vi "+S2C_Omnia8257_Process.vi"(8 "Error In":errorcluster) -> (0 "Error Out":errorcluster)   [LabVIEW 2015]
uses:
  VIs/S2C_OM8257_Proc_Globals.vi
panel:
  out "Err":bool
  in  "Clear":bool
  out "Exit":bool
  in  "LogDepth":u32=10 caption="Log Depth"
  in  "CtrlTab":T1(tab)
  in  "Init":T2={"P1C1"={"Resource Name"="COM4", "Baud Rate"=57600, "Data Bits"=8, "Parity"=0, "Stop Bits"=10, "Flow Control"=0, "Timeout"=5000, "Reset"=TRUE, "P1C1Exe"=FALSE}} {"P1C1"."Parity" items=["None", "Odd", "Even", "Mark", "Space"]; "P1C1"."Flow Control" items=["None", "XON/XOFF", "RTS/CTS", "XON/XOFF & RTS/CTS", "DTR/DSR", "XON/XOFF & DTR/DSR"]; "P1C1"."Stop Bits" items=["1.0"=10, "1.5"=15, "2.0"=20]; "P1C1"."Data Bits" min=7 max=8 step=1}
  in  "CFG-Step":enum32{"ACW", "LLT", "GND", "RUN", "PROMPT"}(tab)
  in  "ACW":T3={"Voltage (V)"=1240, "High Limit Total (mA)"=10.0, "Low Limit Total (mA)"=0.0, "Ramp Up Time (s)"=0.1, "Dwell Time (s)"=1.0, "Arc Sense"=5, "Arc Detect"=FALSE, "High Limit Real (mA)"=10.0, "Low Limit Real (mA)"=0.0, "Ramp Down Time (s)"=0.0, "Continuity"=FALSE, "Offset (mA)"=0.0, "Auto Offset"=FALSE, "DUT Output"=FALSE, "Frequency (Hz)"=60, "Scanner?"=FALSE, "Step Selection"=1, "Add Step"=FALSE, "ACW-Scan"={"Scan16"=1, "Scan15"=1, "Scan14"=1, "Scan13"=1, "Scan12"=1, "Scan11"=1, "Scan10"=1, "Scan9"=1, "Scan8"=1, "Scan7"=1, "Scan6"=1, "Scan5"=1, "Scan4"=1, "Scan3"=1, "Scan2"=1, "Scan1"=1}, "P1P1C1Exe"=FALSE} caption="CfgStep ACW" {"ACW-Scan"."Scan16" min=0 max=2 step=1 scale=0.0..2.0; "ACW-Scan"."Scan15" min=0 max=2 step=1 scale=0.0..2.0; "ACW-Scan"."Scan14" min=0 max=2 step=1 scale=0.0..2.0; "ACW-Scan"."Scan13" min=0 max=2 step=1 scale=0.0..2.0; "ACW-Scan"."Scan12" min=0 max=2 step=1 scale=0.0..2.0; "ACW-Scan"."Scan11" min=0 max=2 step=1 scale=0.0..2.0; "ACW-Scan"."Scan10" min=0 max=2 step=1 scale=0.0..2.0; "ACW-Scan"."Scan9" min=0 max=2 step=1 scale=0.0..2.0; "ACW-Scan"."Scan8" min=0 max=2 step=1 scale=0.0..2.0; "ACW-Scan"."Scan7" min=0 max=2 step=1 scale=0.0..2.0; "ACW-Scan"."Scan6" min=0 max=2 step=1 scale=0.0..2.0; "ACW-Scan"."Scan5" min=0 max=2 step=1 scale=0.0..2.0; "ACW-Scan"."Scan4" min=0 max=2 step=1 scale=0.0..2.0; "ACW-Scan"."Scan3" min=0 max=2 step=1 scale=0.0..2.0; "ACW-Scan"."Scan2" min=0 max=2 step=1 scale=0.0..2.0; "ACW-Scan"."Scan1" min=0 max=2 step=1 scale=0.0..2.0; "Offset (mA)" format="%.2g"; "Ramp Down Time (s)" format="%.1g"; "Dwell Time (s)" format="%.1g"; "High Limit Real (mA)" format="%.2g"; "Low Limit Total (mA)" format="%.3g"; "High Limit Total (mA)" format="%.2g"; "Low Limit Real (mA)" format="%.3g"; "Ramp Up Time (s)" format="%.1g"}
  in  "LLT":T4={"Leakage-Hi (V)"=6000.0, "Leakage-Lo (V)"=0.0, "Voltage-Hi (V)"=125.0, "Voltage-Lo (V)"=0.0, "Dwell (s)"=0.5, "Delay (s)"=1.0, "Offset (uA)"=10.0, "AC Src Voltage (V)"=115.0, "AC Src A-Hi (A)"=0.0, "AC Source"=FALSE, "AC Src Frequency"=60.0, "Auto Offset"=FALSE, "Reverse"=FALSE, "Active Link"=FALSE, "AC Src OC Fold"=FALSE, "Neutral"=FALSE, "Ground"=FALSE, "Leakage"=FALSE, "Ranging Mode"=FALSE, "AC Src Output"=TRUE, "AC Src Range"=TRUE, "Measure Device"=0, "Probe"=0, "Filter Mode"=0, "Scanner?"=FALSE, "Step Selection"=1, "Add Step"=FALSE, "ACW-Scan"={"Scan16"=1, "Scan15"=1, "Scan14"=1, "Scan13"=1, "Scan12"=1, "Scan11"=1, "Scan10"=1, "Scan9"=1, "Scan8"=1, "Scan7"=1, "Scan6"=1, "Scan5"=1, "Scan4"=1, "Scan3"=1, "Scan2"=1, "Scan1"=1}, "P1P2C1Exe"=FALSE} caption="CfgStep LLT" {"Filter Mode" items=["AC+DC", "AC", "DC"]; "Probe" items=["Ground To Line", "Probe-HI To Line", "Probe-HI To Probe-Lo"]; "Measure Device" items=["UL544NP", "UL544P", "IEC60601 UL2601", "UL1563", "IEC60990 Fig4-U1 IEC60950", "IEC60990 Fig4-U2 IEC60950", "IEC60990 Fig5-U3", "External", "N/A", "Frequency Check"]; "AC Src Frequency" format="%#.6f"; "Offset (uA)" format="%#.2g"; "ACW-Scan"."Scan16" min=0 max=2 step=1 scale=0.0..2.0; "ACW-Scan"."Scan15" min=0 max=2 step=1 scale=0.0..2.0; "ACW-Scan"."Scan14" min=0 max=2 step=1 scale=0.0..2.0; "ACW-Scan"."Scan13" min=0 max=2 step=1 scale=0.0..2.0; "ACW-Scan"."Scan12" min=0 max=2 step=1 scale=0.0..2.0; "ACW-Scan"."Scan11" min=0 max=2 step=1 scale=0.0..2.0; "ACW-Scan"."Scan10" min=0 max=2 step=1 scale=0.0..2.0; "ACW-Scan"."Scan9" min=0 max=2 step=1 scale=0.0..2.0; "ACW-Scan"."Scan8" min=0 max=2 step=1 scale=0.0..2.0; "ACW-Scan"."Scan7" min=0 max=2 step=1 scale=0.0..2.0; "ACW-Scan"."Scan6" min=0 max=2 step=1 scale=0.0..2.0; "ACW-Scan"."Scan5" min=0 max=2 step=1 scale=0.0..2.0; "ACW-Scan"."Scan4" min=0 max=2 step=1 scale=0.0..2.0; "ACW-Scan"."Scan3" min=0 max=2 step=1 scale=0.0..2.0; "ACW-Scan"."Scan2" min=0 max=2 step=1 scale=0.0..2.0; "ACW-Scan"."Scan1" min=0 max=2 step=1 scale=0.0..2.0; "Voltage-Lo (V)" format="%#.2g"; "Voltage-Hi (V)" format="%#.3g"; "Leakage-Lo (V)" format="%#.2g"; "Dwell (s)" format="%.1g"}
  in  "GND":T5={"Current (A)"=1240.0, "Voltage (V)"=10.0, "Hi-Limit (mohm)"=100, "Lo-Limit (mhom)"=0, "Dwell (s)"=1.0, "Offset (mhom)"=0, "Auto Offset"=FALSE, "Frequency (Hz)"=60, "DualCHEK"=0, "Scanner Selection"=0, "Scanner?"=FALSE, "Step Selection"=1, "Add Step"=FALSE, "P1P3C1Exe"=FALSE} caption="CfgStep GND" {"DualCHEK" items=["OFF", "ACW", "DCW"]}
  in  "RUN":T6={"Voltage-Hi (V)"=125.0, "Voltage-Lo (V)"=0.0, "Amp-Hi (A)"=10.0, "Amp-Lo (A)"=0.0, "Dwell (s)"=1.0, "Delay (s)"=0.2, "Leakage-Hi (mA)"=10.0, "Leakage-Lo (mA)"=0.0, "Power-Hi (W)"=1000, "Power-Lo (W)"=0, "PF-Hi"=1.0, "PF-Lo"=0.0, "AC Src Voltage (V)"=115.0, "AC Src A-Hi (A)"=0.0, "AC Source"=FALSE, "AC Src Frequency (Hz)"=60, "AC Src OC Fold"=FALSE, "AC Src Output"=TRUE, "AC Src Range"=TRUE, "Active Link"=FALSE, "Step Selection"=1, "Add Step"=FALSE, "P1P4C1Exe"=FALSE} caption="CfgStep RUN"
  in  "Prompt":cluster{"Prompt":string, "P1P5C1Exe":bool}={"Prompt"="<Enter Prompt>", "P1P5C1Exe"=FALSE} caption="CfgStep Prompt"
  in  "CfgSys":T7
  in  "ActStatus":cluster{"P4C1":cluster{"P4C1Exe":bool}}
  in  "ActFile":T8={"P5C1"={"File Number"=1, "Filename"="<Filename>", "P5C1Exe"=FALSE}, "P5C2"={"File Number"=1, "P5C2Exe"=FALSE}, "P5C3"={"File Number"=1, "P5C3Exe"=FALSE}, "P5C4"={"File Number"=1, "P5C4Exe"=FALSE}, "P5C5"={"Fail Stop"=FALSE, "P5C5Exe"=FALSE}}
  in  "ActStep":cluster{"P6C1":cluster{"P6C1Exe":bool}}
  in  "DataLL":T9={"P7C1"={"Result Number"=1, "P7C1Exe"=FALSE}, "P7C2"={"P7C2Exe"=FALSE}}
  in  "Utility":cluster{"P8C1":cluster{"P8C1Exe":bool}}
  in  "CommLog":string caption="Communication Log"
  # "Main Cluster:\n394x886\n1 = 355x876\n2 = 355x438\n3 = 355x292\n4 = 163x438\n6 = 163x292\n8 = 163x219 \n\nSubTab 369x886\nSubClust 359x876"
  # "Omina II 8257 Driver Panel"
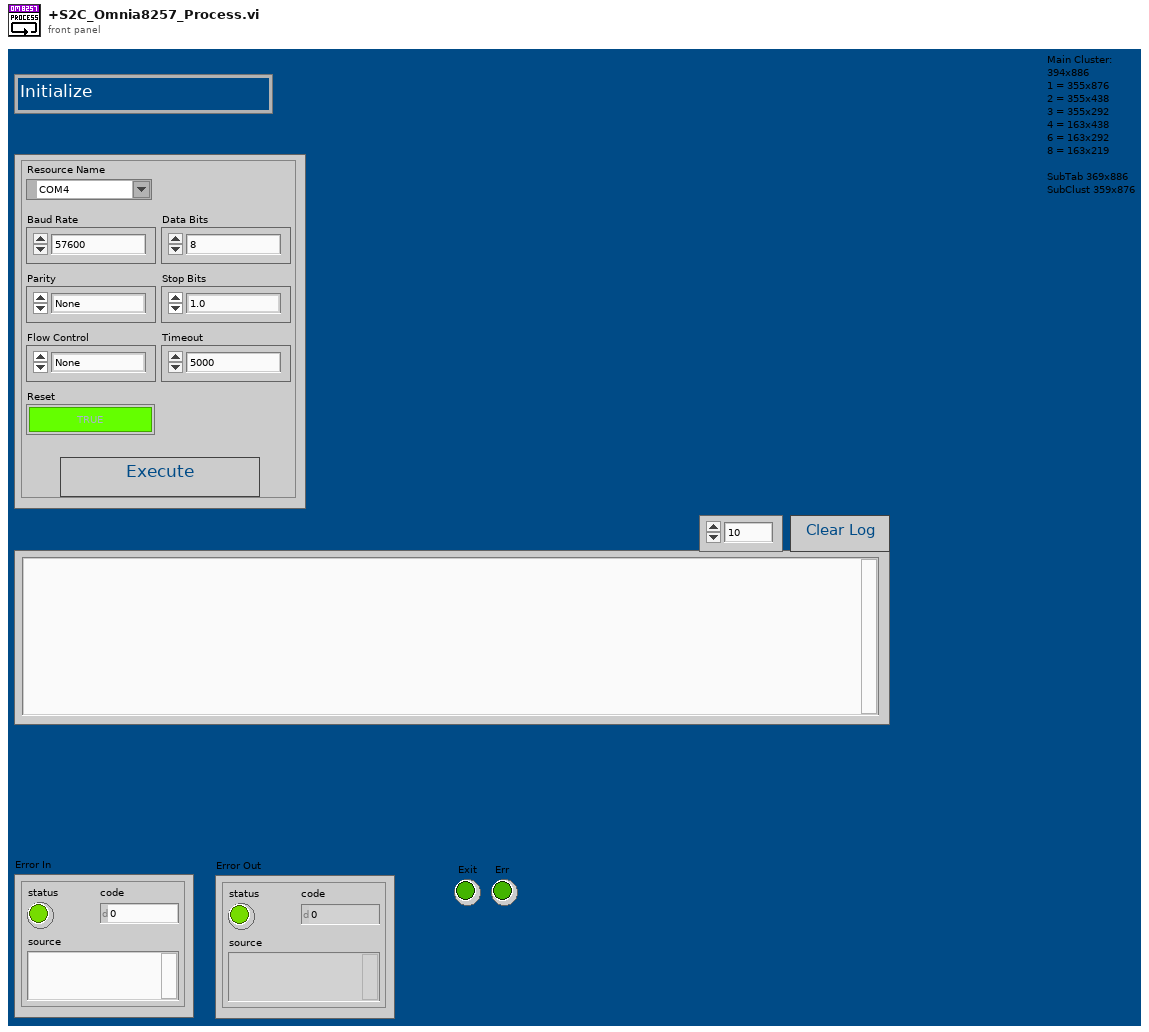
[diagram p1: front panel]
types:
  T1 = enum32{"Initialize", "Cfg:Step", "Cfg:System", "Act-Status", "Act-Stat:File", "Act-Stat:Step", "Data:Low Level", "Utility"}
  T2 = cluster{"P1C1":cluster{"Resource Name":refnum<visa-resource-name>, "Baud Rate":u32, "Data Bits":u16, "Parity":u16, "Stop Bits":u16, "Flow Control":u16, "Timeout":u32, "Reset":bool, "P1C1Exe":bool}}
  T3 = cluster{"Voltage (V)":u16, "High Limit Total (mA)":dbl, "Low Limit Total (mA)":dbl, "Ramp Up Time (s)":dbl, "Dwell Time (s)":dbl, "Arc Sense":u8, "Arc Detect":bool, "High Limit Real (mA)":dbl, "Low Limit Real (mA)":dbl, "Ramp Down Time (s)":dbl, "Continuity":bool, "Offset (mA)":dbl, "Auto Offset":bool, "DUT Output":bool, "Frequency (Hz)":u16, "Scanner?":bool, "Step Selection":i32, "Add Step":bool, "ACW-Scan":cluster{"Scan16":i32, "Scan15":i32, "Scan14":i32, "Scan13":i32, "Scan12":i32, "Scan11":i32, "Scan10":i32, "Scan9":i32, "Scan8":i32, "Scan7":i32, "Scan6":i32, "Scan5":i32, "Scan4":i32, "Scan3":i32, "Scan2":i32, "Scan1":i32}, "P1P1C1Exe":bool}
  T4 = cluster{"Leakage-Hi (V)":dbl, "Leakage-Lo (V)":dbl, "Voltage-Hi (V)":dbl, "Voltage-Lo (V)":dbl, "Dwell (s)":dbl, "Delay (s)":dbl, "Offset (uA)":dbl, "AC Src Voltage (V)":dbl, "AC Src A-Hi (A)":dbl, "AC Source":bool, "AC Src Frequency":dbl, "Auto Offset":bool, "Reverse":bool, "Active Link":bool, "AC Src OC Fold":bool, "Neutral":bool, "Ground":bool, "Leakage":bool, "Ranging Mode":bool, "AC Src Output":bool, "AC Src Range":bool, "Measure Device":u16, "Probe":u16, "Filter Mode":u16, "Scanner?":bool, "Step Selection":i32, "Add Step":bool, "ACW-Scan":cluster{"Scan16":i32, "Scan15":i32, "Scan14":i32, "Scan13":i32, "Scan12":i32, "Scan11":i32, "Scan10":i32, "Scan9":i32, "Scan8":i32, "Scan7":i32, "Scan6":i32, "Scan5":i32, "Scan4":i32, "Scan3":i32, "Scan2":i32, "Scan1":i32}, "P1P2C1Exe":bool}
  T5 = cluster{"Current (A)":dbl, "Voltage (V)":dbl, "Hi-Limit (mohm)":u16, "Lo-Limit (mhom)":u16, "Dwell (s)":dbl, "Offset (mhom)":u16, "Auto Offset":bool, "Frequency (Hz)":u16, "DualCHEK":u16, "Scanner Selection":i32, "Scanner?":bool, "Step Selection":i32, "Add Step":bool, "P1P3C1Exe":bool}
  T6 = cluster{"Voltage-Hi (V)":dbl, "Voltage-Lo (V)":dbl, "Amp-Hi (A)":dbl, "Amp-Lo (A)":dbl, "Dwell (s)":dbl, "Delay (s)":dbl, "Leakage-Hi (mA)":dbl, "Leakage-Lo (mA)":dbl, "Power-Hi (W)":u16, "Power-Lo (W)":u16, "PF-Hi":dbl, "PF-Lo":dbl, "AC Src Voltage (V)":dbl, "AC Src A-Hi (A)":dbl, "AC Source":bool, "AC Src Frequency (Hz)":u16, "AC Src OC Fold":bool, "AC Src Output":bool, "AC Src Range":bool, "Active Link":bool, "Step Selection":i32, "Add Step":bool, "P1P4C1Exe":bool}
  T7 = cluster{"P3C1":cluster{"DUT HV":bool, "P3C1Exe":bool}}
  T8 = cluster{"P5C1":cluster{"File Number":i32, "Filename":string, "P5C1Exe":bool}, "P5C2":cluster{"File Number":u16, "P5C2Exe":bool}, "P5C3":cluster{"File Number":u16, "P5C3Exe":bool}, "P5C4":cluster{"File Number":u16, "P5C4Exe":bool}, "P5C5":cluster{"Fail Stop":bool, "P5C5Exe":bool}}
  T9 = cluster{"P7C1":cluster{"Result Number":i32, "P7C1Exe":bool}, "P7C2":cluster{"P7C2Exe":bool}}
  T10 = cluster{"Caller-Q":refnum<queue>, "Command":string, "Return":string, "Data":variant, "Timeout":dbl}
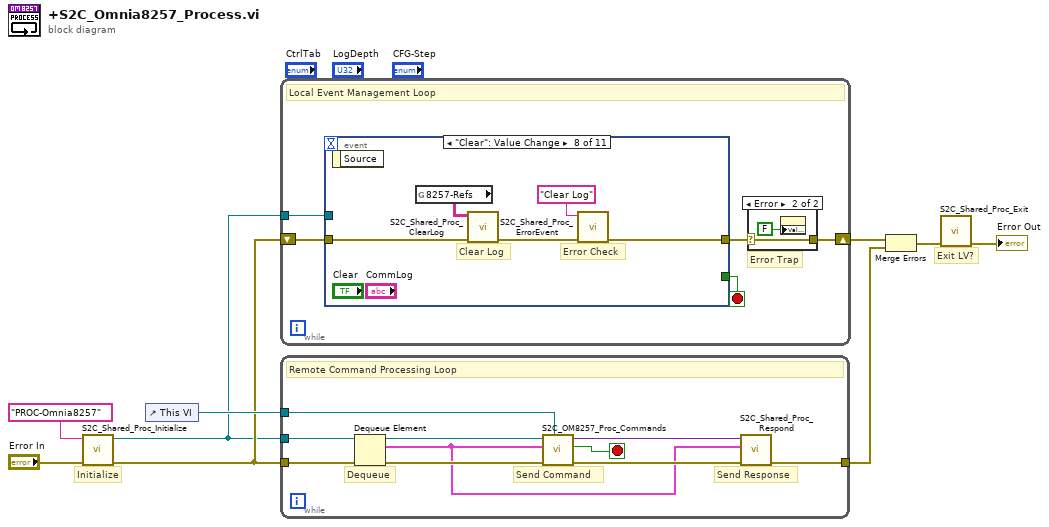
[diagram p0: block diagram]
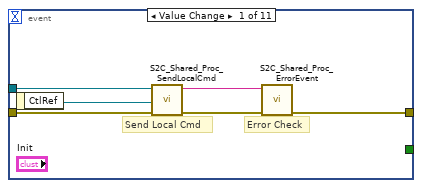
[diagram p3: hidden frame]
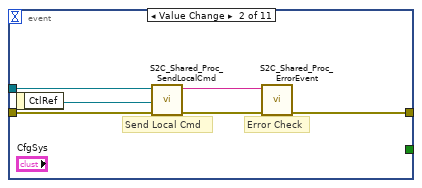
[diagram p4: hidden frame]
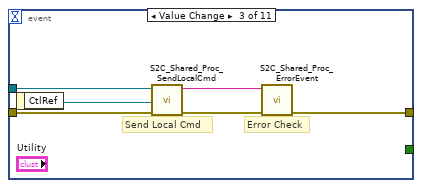
[diagram p5: hidden frame]
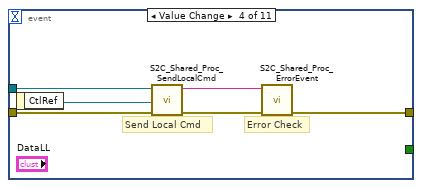
[diagram p6: hidden frame]
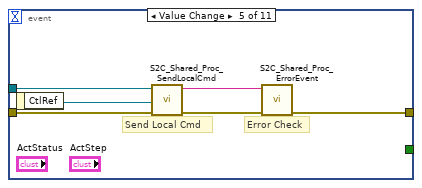
[diagram p7: hidden frame]
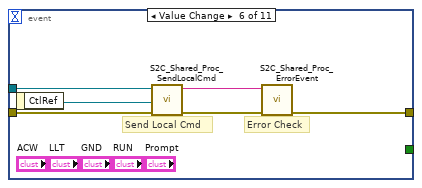
[diagram p8: hidden frame]
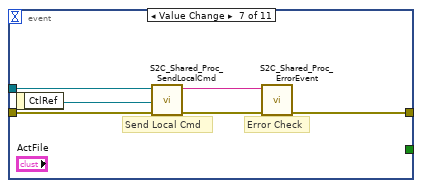
[diagram p9: hidden frame]
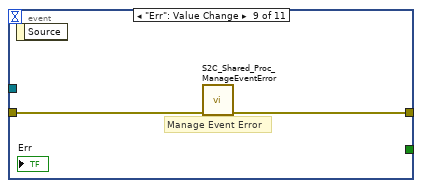
[diagram p10: hidden frame]
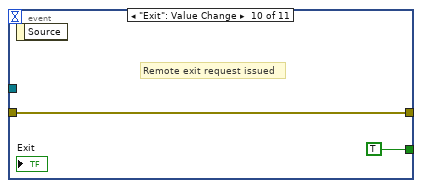
[diagram p11: hidden frame]
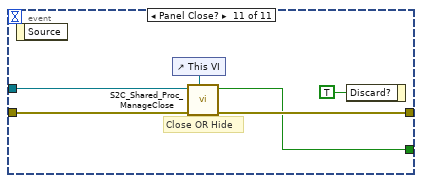
[diagram p12: hidden frame]
diagram:
  # "Exit LV?"
  # "Initialize"
  n1 = call "S2C_Shared_Proc_Initialize.vi"("Error In"="Error In", "Q-Name"="PROC-Omnia8257" ("name (unnamed)")) -> ("Error Out"=w4:errorcluster, "Q-Ref"=w1:refnum<queue>)  [unwired: 8 in]
  n2 = control-ref of="This VI"() -> (w5:refnum<vi>)
  n3 = while {
    tunnel: w1 -> [w12]
    shift-right: [w10] -> w7
    shift-left: w4 -> [w14]
    stop <- w13 stop-if-true
    # "Error Trap"
    # "Local Event Management Loop"
    n4 = event shown="[7] \"Clear\": Value Change" {
      selector: _ -> [_ _ _ _ _ _ _ _ _ _ _]
      dyn-events: _ -> [_ _ _ _ _ _ _ _ _ _ _]
      timeout: _ -> [_ _ _ _ _ _ _ _ _ _ _]
      tunnel: w14 -> [w23 w29 w35 w41 w47 w53 w59 w64 w66 w68 w73]
      tunnel: w12 -> [w21 w27 w33 w39 w45 w51 w57 _ _ _ w71]
      tunnel: [w19 w25 w31 w37 w42 w49 w55 w61 w65 w68 w72] -> w11
      tunnel: [_ _ _ _ _ _ _ _ _ TRUE ("Discard?") w70] -> w13
      event "Init.P1C1.P1C1Exe": Value Change {
        # "Error Check"
        # "Send Local Cmd"
        n5 = event-data() -> ("CtlRef"=w22:refnum<vi>)  [unwired: 1 in]
        n6 = call "S2C_Shared_Proc_SendLocalCmd.vi"("Error In"=w23, "ExeRef"=w22, "Q-Ref"=w21) -> ("Error Out"=w20:errorcluster, "Command"=w18:string)  [unwired: 7 in]
        n7 = call "S2C_Shared_Proc_ErrorEvent.vi"("Error In"=w20, "Command"=w18) -> ("Error Out"=w19:errorcluster)  [unwired: 9 in]
      }
      event "CfgSys.P3C1.P3C1Exe": Value Change {
        # "Error Check"
        # "Send Local Cmd"
        n8 = event-data() -> ("CtlRef"=w28:refnum<vi>)  [unwired: 1 in]
        n9 = call "S2C_Shared_Proc_SendLocalCmd.vi"("Error In"=w29, "ExeRef"=w28, "Q-Ref"=w27) -> ("Error Out"=w26:errorcluster, "Command"=w24:string)  [unwired: 7 in]
        n10 = call "S2C_Shared_Proc_ErrorEvent.vi"("Error In"=w26, "Command"=w24) -> ("Error Out"=w25:errorcluster)  [unwired: 9 in]
      }
      event "Utility.P8C1.P8C1Exe": Value Change {
        # "Error Check"
        # "Send Local Cmd"
        n11 = event-data() -> ("CtlRef"=w34:refnum<vi>)  [unwired: 1 in]
        n12 = call "S2C_Shared_Proc_SendLocalCmd.vi"("Error In"=w35, "ExeRef"=w34, "Q-Ref"=w33) -> ("Error Out"=w32:errorcluster, "Command"=w30:string)  [unwired: 7 in]
        n13 = call "S2C_Shared_Proc_ErrorEvent.vi"("Error In"=w32, "Command"=w30) -> ("Error Out"=w31:errorcluster)  [unwired: 9 in]
      }
      event "DataLL.P7C1.P7C1Exe", "DataLL.P7C2.P7C2Exe": Value Change {
        # "Error Check"
        # "Send Local Cmd"
        n14 = event-data() -> ("CtlRef"=w40:refnum<vi>)  [unwired: 1 in]
        n15 = call "S2C_Shared_Proc_SendLocalCmd.vi"("Error In"=w41, "ExeRef"=w40, "Q-Ref"=w39) -> ("Error Out"=w38:errorcluster, "Command"=w36:string)  [unwired: 7 in]
        n16 = call "S2C_Shared_Proc_ErrorEvent.vi"("Error In"=w38, "Command"=w36) -> ("Error Out"=w37:errorcluster)  [unwired: 9 in]
      }
      event "ActStatus.P4C1.P4C1Exe", "ActStep.P6C1.P6C1Exe": Value Change {
        # "Error Check"
        # "Send Local Cmd"
        n17 = event-data() -> ("CtlRef"=w46:refnum<vi>)  [unwired: 1 in]
        n18 = call "S2C_Shared_Proc_SendLocalCmd.vi"("Error In"=w47, "ExeRef"=w46, "Q-Ref"=w45) -> ("Error Out"=w44:errorcluster, "Command"=w43:string)  [unwired: 7 in]
        n19 = call "S2C_Shared_Proc_ErrorEvent.vi"("Error In"=w44, "Command"=w43) -> ("Error Out"=w42:errorcluster)  [unwired: 9 in]
      }
      event "ACW.P1P1C1Exe", "LLT.P1P2C1Exe", "GND.P1P3C1Exe", "RUN.P1P4C1Exe", "Prompt.P1P5C1Exe": Value Change {
        # "Error Check"
        # "Send Local Cmd"
        n20 = event-data() -> ("CtlRef"=w52:refnum<vi>)  [unwired: 1 in]
        n21 = call "S2C_Shared_Proc_SendLocalCmd.vi"("Error In"=w53, "ExeRef"=w52, "Q-Ref"=w51) -> ("Error Out"=w50:errorcluster, "Command"=w48:string)  [unwired: 7 in]
        n22 = call "S2C_Shared_Proc_ErrorEvent.vi"("Error In"=w50, "Command"=w48) -> ("Error Out"=w49:errorcluster)  [unwired: 9 in]
      }
      event "ActFile.P5C1.P5C1Exe", "ActFile.P5C2.P5C2Exe", "ActFile.P5C3.P5C3Exe", "ActFile.P5C4.P5C4Exe", "ActFile.P5C5.P5C5Exe": Value Change {
        # "Error Check"
        # "Send Local Cmd"
        n23 = event-data() -> ("CtlRef"=w58:refnum<vi>)  [unwired: 1 in]
        n24 = call "S2C_Shared_Proc_SendLocalCmd.vi"("Error In"=w59, "ExeRef"=w58, "Q-Ref"=w57) -> ("Error Out"=w56:errorcluster, "Command"=w54:string)  [unwired: 7 in]
        n25 = call "S2C_Shared_Proc_ErrorEvent.vi"("Error In"=w56, "Command"=w54) -> ("Error Out"=w55:errorcluster)  [unwired: 9 in]
      }
      event "Clear": Value Change {
        # "Error Check"
        # "Clear Log"
        n26 = event-data() -> ()  [unwired: 1 in, 1 out]
        n27 = global read "S2C_OM8257_Proc_Globals.vi" "8257-Refs"() -> (w63:string[][])
        n28 = call "S2C_Shared_Proc_ClearLog.vi"("Error In"=w64, "Refs"=w63) -> ("Error Out"=w62:errorcluster)  [unwired: 9 in]
        n29 = call "S2C_Shared_Proc_ErrorEvent.vi"("Error In"=w62, "Command"="Clear Log") -> ("Error Out"=w61:errorcluster)  [unwired: 9 in]
      }
      event "Err": Value Change {
        # "Manage Event Error"
        n30 = event-data() -> ()  [unwired: 1 in, 1 out]
        n31 = call "S2C_Shared_Proc_ManageEventError.vi"("Error In"=w66) -> ("Error Out"=w65:errorcluster)  [unwired: 10 in]
      }
      event "Exit": Value Change {
        # "Remote exit request issued"
        n32 = event-data() -> ()  [unwired: 1 in, 1 out]
      }
      event Panel Close? {
        # "Close OR Hide"
        n33 = event-data() -> ()  [unwired: 1 in, 1 out]
        n34 = control-ref of="This VI"() -> (w69:refnum<vi>)
        n35 = call "S2C_Shared_Proc_ManageClose.vi"("VI_Ref"=w69, "Error In"=w73, "Q-Ref"=w71) -> ("Error Out"=w72:errorcluster, "Exit?"=w70:bool)  [unwired: 7 in]
        n36 = event-data("Discard?"=TRUE) -> ()  [unwired: 1 in, 1 out]
      }
    }
    n37 = case shown="Error" w11 {
      selector: w11 -> [w15 w16]
      tunnel: [w15 w16] -> w10
      frame No Error {
      }
      frame Error {
        n38 = property on="Err" class="Bool (strict)"("Val(Sgnl)"=FALSE ("Value (Signaling)")) -> ()  [unwired: 2 in, 2 out]
      }
    }
  }
  n39 = while {
    tunnel: w1 -> [w77]
    tunnel: w5 -> [w79]
    tunnel: w4 -> [w84]
    tunnel: [w78] -> w6
    stop <- w80 stop-if-true
    # "Send Response"
    # "Send Command"
    # "Dequeue"
    # "Remote Command Processing Loop"
    n40 = Dequeue Element(queue=w77, error in (no error)=w84) -> (queue out=w76:refnum<queue>, element=w75:T10, error out=w83:errorcluster)  [unwired: 1 in, 1 out]
    n41 = call "S2C_OM8257_Proc_Commands.vi"("VI_Ref"=w79, "Error In"=w83, "Settings"=w75, "Q-Ref"=w76) -> ("Error Out"=w81:errorcluster, "Stop?"=w80:bool, "Response"=w82:variant)  [unwired: 5 in]
    n42 = call "S2C_Shared_Proc_Respond.vi"("Error In"=w81, "Settings"=w75, "Response"=w82) -> ("Error Out"=w78:errorcluster)  [unwired: 8 in]
  }
  n43 = Merge Errors(w7, w6) -> (w3:errorcluster)
  n44 = call "S2C_Shared_Proc_Exit.vi"("Error In"=w3) -> ("Error Out"=→"Error Out":errorcluster)  [unwired: 10 in]
